vi "Append Section to HHP.vi"(10 "Value":string, 11 "HHP String In":string) -> (3 "HHP String Out":string)   [LabVIEW 2015, in "CHM Generator.lvclass"]
uses:
  CHM Generator.lvclass
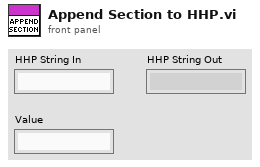
[diagram p1: front panel]
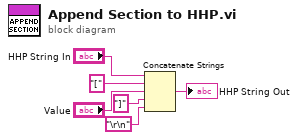
[diagram p0: block diagram]
diagram:
  n1 = Concatenate Strings("HHP String In", "[" ("string"), "Value", "]" ("string"), "\r\n") -> (→"HHP String Out":string)
